vi "MC5e List Squds in Unit Strings.vi"(11 "Unit index":i32) -> (3 "Squad Strings":string[](array[string]))   [LabVIEW 2020]
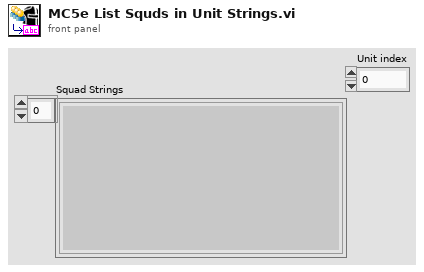
[diagram p1: front panel]
types:
  T1 = typedef "MC5e Unit.ctl" = cluster{"Unit Fatigue Level":enum16{"Not Fatigued", "Fatigued", "Seriously Fatigued"}, "Flying Unit":bool, "Mounted Unit":bool, "Defending from Stronghold":bool, "Difficult Terrain Types":T2, "Squads in Unit":T3[], "Unit Info":T5, "Range":i32, "BR":i32, "Speed":i32, "Morale":i32, "Current BR":i32, "Location":T6, "Capacity %":i32}
  T2 = typedef "MC5e Terrain types.ctl" = i32[]
  T3 = typedef "MC5e Squad_Info.ctl" = cluster{"Squad Name":string, "# Soldiers":u16, "Battle Rating":u16, "Flying":bool, "Mounted":bool, "Speed":u16, "Range":u16, "Morale":i32, "Max Endurance":u16, "Current Endurance":i32, "Size":T4, "Space Taken":u16, "Difficult Terrain":i32[], "CR":u16, "Special / Notes":string}
  T4 = typedef "MC5e Size_Categories.ctl" = enum16{"Tiny", "Small", "Medium", "Large", "Huge", "Gargantuan"}
  T5 = typedef "MC5e Unit Header.ctl" = cluster{"Unit Name":string, "Unit Commander":string, "Morale Mod":i32, "BR Mod":i32, "Defense Mod":i32, "Speed Mod":i32, "Unit Notes":string, "Attack Mod":i32, "Unit Wins+ Losses-":i32, "Commander Charisma Bonus":i32}
  T6 = typedef "Location.ctl" = cluster{"X coordinate":dbl, "Y coordinate":dbl}
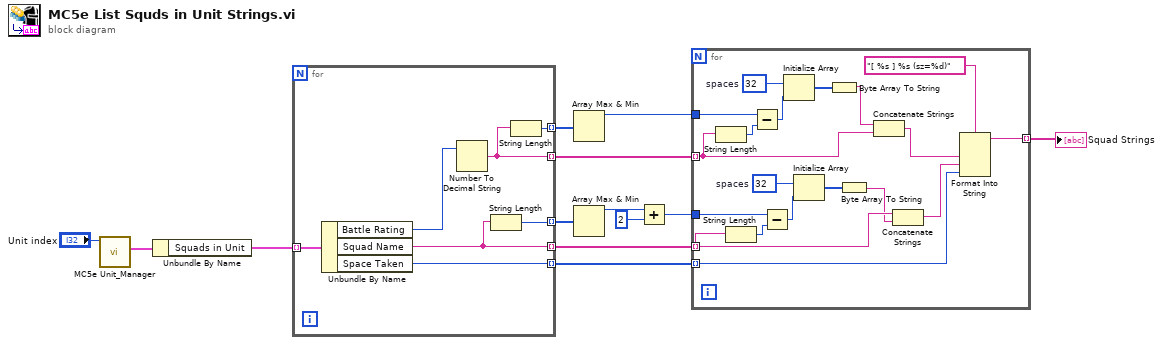
[diagram p0: block diagram]
diagram:
  n1 = call "MC5e Unit_Manager.vi"("index (get/delete)"="Unit index") -> ("Unit"=w2:T1)  [unwired: 7 in, 3 out]
  n2 = Unbundle By Name(w2) -> ("Squads in Unit"=w1:T3[])
  n3 = for {
    tunnel: [w16] -> w10 mode=indexing
    tunnel: [w20] -> w13 mode=indexing
    tunnel: [w15] -> w8 mode=indexing
    tunnel: [w19] -> w9 mode=indexing
    tunnel: [w18] -> w4 mode=indexing
    tunnel: w1 -> [w14] mode=indexing
    n4 = Unbundle By Name(w14) -> ("Battle Rating"=w17:u16, "Squad Name"=w16:string, "Space Taken"=w15:u16)
    n5 = Number To Decimal String(number=w17) -> (decimal integer string=w19:string)  [unwired: 1 in]
    n6 = String Length(string=w16) -> (length=w20:i32)
    n7 = String Length(string=w19) -> (length=w18:i32)
  }
  n8 = Array Max & Min(array=w4) -> (max value=w5:i32)  [unwired: 3 out]
  n9 = Array Max & Min(array=w13) -> (max value=w12:i32)  [unwired: 3 out]
  n10 = Add(x=w12, y=2) -> (x+y=w6:i32)
  n11 = for {
    tunnel: w10 -> [w31] mode=indexing
    tunnel: w9 -> [w23] mode=indexing
    tunnel: w8 -> [w38] mode=indexing
    tunnel: [w37] -> w7 mode=indexing
    tunnel: w6 -> [w35]
    tunnel: w5 -> [w24]
    w27 = u8 32  # spaces
    w33 = u8 32  # spaces
    n12 = String Length(string=w23) -> (length=w25:i32)
    n13 = String Length(string=w31) -> (length=w36:i32)
    n14 = Subtract(x=w24, y=w25) -> (x-y=w28:i32)
    n15 = Subtract(x=w35, y=w36) -> (x-y=w32:i32)
    n16 = Initialize Array(w27, w28) -> (w26:u8[])
    n17 = Initialize Array(w33, w32) -> (w34:u8[])
    n18 = Byte Array To String(unsigned byte array=w26) -> (string=w22:string)
    n19 = Byte Array To String(unsigned byte array=w34) -> (string=w30:string)
    n20 = Concatenate Strings(w22, w23) -> (w21:string)
    n21 = Concatenate Strings(w31, w30) -> (w29:string)
    n22 = Format Into String(format string="[ %s ] %s (sz=%d)", w21, w29, w38) -> (resulting string=w37:string)  [unwired: 2 in, 1 out]
  }
  "Squad Strings" <- w7
